vi "Calculate Pump Head-Flow Curves.vi"(6 "Points (100)":i32=100, 8 "n":dbl=4.278 format="%#_13g", 9 "A":dbl=5.216e-06 format="%#_13g", 10 "Shut-off head":dbl=320.0 format="%#_13g", 11 "Run-out flow":dbl=50.0 format="%#_13g") -> (2 "head":dbl[](array[numeric]), 3 "flow":dbl[](array[numeric]))   [LabVIEW 2020]
doc: "Calculates head-flow curves for a pump or compressor using an equation in the form of \"head= shut-off head - A * flow^n\" based on the shut-off head, run-out flow, and values for the coefficient \"A\" and exponent \"n.\" Any unit set can be used for flow and head as long as the coefficient and exponent values are consistent."
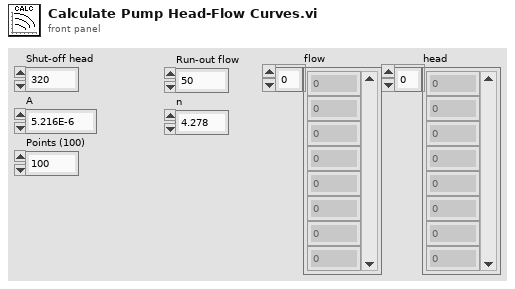
[diagram p1: front panel]
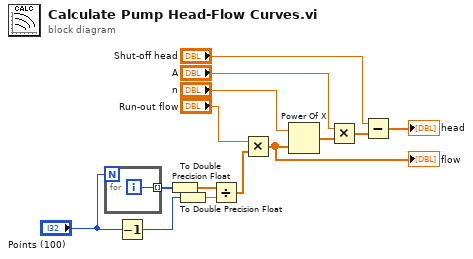
[diagram p0: block diagram]
diagram:
  n1 = for {
    N: "Points (100)" -> [_]
    tunnel: [w15] -> w1 mode=indexing
    i -> [w15]
  }
  n2 = Decrement(x="Points (100)") -> (x-1=w14:i32)
  n3 = To Double Precision Float(number=w1) -> (double precision float=w3:dbl[])
  n4 = To Double Precision Float(number=w14) -> (double precision float=w4:dbl)
  n5 = Divide(x=w3, y=w4) -> (x/y=w5:dbl[])
  n6 = Multiply(x="Run-out flow", y=w5) -> (x*y=w13:dbl[])
  "flow" <- w13
  n7 = Power Of X(1:w13, 2:"n") -> (0:w8:dbl[])
  n8 = Multiply(x="A", y=w8) -> (x*y=w10:dbl[])
  n9 = Subtract(x="Shut-off head", y=w10) -> (x-y=→"head":dbl[])
